vi "niRFSTS Digital Configure PPMU.vi"(0 "Semiconductor Module Context":T2, 3 "aperture time":dbl=4e-06 format="%#_6p", 4 "Level (V or A)":dbl, 5 "Pin Names":string[](array[string]), 9 "output function":T1=1300 items=["DC Voltage"=1300, "DC Current"=1301], 11 "error in (no error)":errorcluster, 12 "voltage limit high":dbl, 14 "voltage limit low":dbl) -> (15 "error out":errorcluster)   [LabVIEW 2014]
uses:
  <vilib>/NI_TestStand_SemiconductorModule/NI_TestStand_Semiconductor_Module.lvlibp/PinMap/General/SemiconductorModuleContext.ctl
  <instrlib>/niDigital/niDigital.llb/niDigital Output Function.ctl
  <instrlib>/niDigital/niDigital.llb/niDigital Selected Function.ctl
  <instrlib>/niDigital/niDigital.llb/niDigital PMU Aperture Time Units.ctl
  <vilib>/NI_TestStand_SemiconductorModule/NI_TestStand_Semiconductor_Module.lvlibp/PinMap/Digital Pattern/PinsToNIDigitalPatternSessions.vi
  <vilib>/NI_TestStand_SemiconductorModule/NI_TestStand_Semiconductor_Module.lvlibp
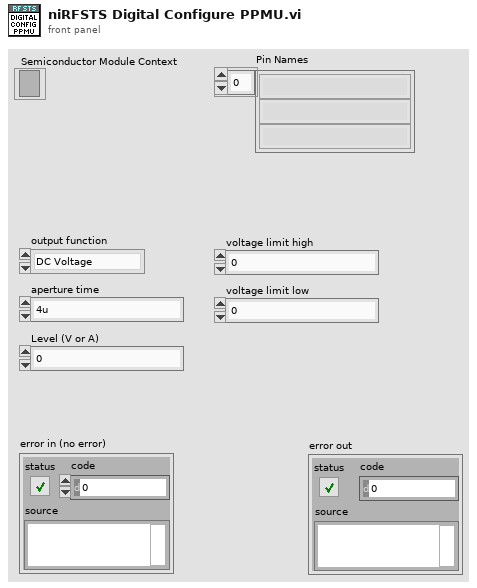
[diagram p1: front panel]
types:
  T1 = typedef "niDigital Output Function.ctl" = i32
  T2 = typedef "NI_TestStand_Semiconductor_Module.lvlibp/SemiconductorModuleContext.ctl" = refnum<k7>
  T3 = typedef "niDigital PMU Aperture Time Units.ctl" = i32
  T4 = typedef "niDigital Selected Function.ctl" = i32
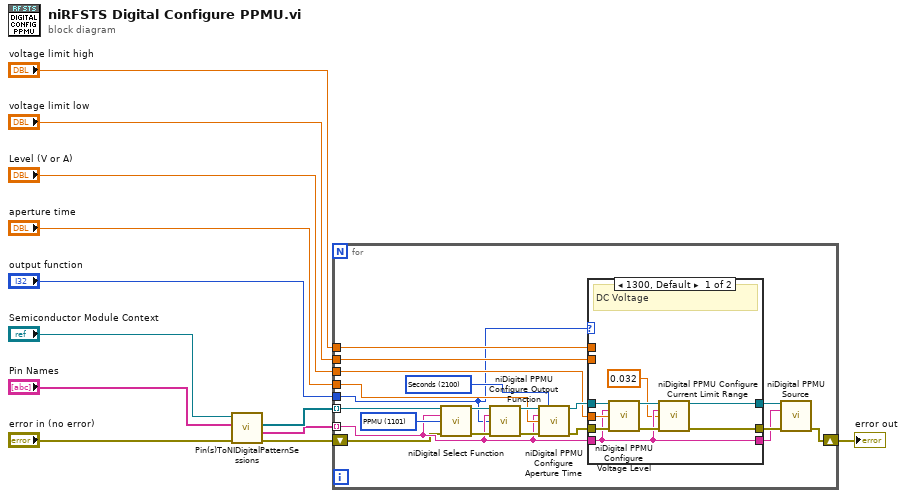
[diagram p0: block diagram]
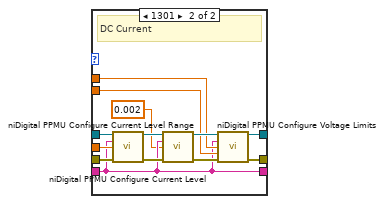
[diagram p2: hidden frame]
diagram:
  n1 = call-poly <vilib>:"Pin(s)ToNIDigitalPatternSessions.vi"("error in (no error)"="error in (no error)", "Pins"="Pin Names", "Semiconductor Module Context"="Semiconductor Module Context") -> ("error out"=w2:errorcluster, "Channel Lists"=w10:string[], "Instrument Sessions"=w11:refnum<k15>[])  [unwired: 3 in, 3 out]
  n2 = for {
    tunnel: w11 -> [w19] mode=indexing
    tunnel: w10 -> [w20] mode=indexing
    tunnel: "output function" -> [w13]
    tunnel: "Level (V or A)" -> [w25]
    tunnel: "voltage limit high" -> [w24]
    tunnel: "voltage limit low" -> [w23]
    tunnel: "aperture time" -> [w22]
    shift-right: [w16] -> w1
    shift-left: w2 -> [w18]
    w21 = T3 2100 items=["Seconds"=2100] ("aperture time units")
    w32 = T4 1101 items=["Digital"=1100, "PPMU"=1101, "Off"=1102, "Disconnect"=1103] ("function")
    n3 = call <instrlib>:"niDigital Select Function.vi"("instrument handle"=w19, "channel list"=w20, "function"=w32, "error in"=w18) -> ("instrument handle out"=w31:refnum<k15>, "error out"=w30:errorcluster)  [unwired: 10 in]
    n4 = call <instrlib>:"niDigital PPMU Configure Output Function.vi"("instrument handle"=w31, "channel list"=w20, "output function"=w13, "error in"=w30) -> ("instrument handle out"=w26:refnum<k15>, "error out"=w29:errorcluster)  [unwired: 10 in]
    n5 = call <instrlib>:"niDigital PPMU Configure Aperture Time.vi"("instrument handle"=w26, "aperture time units"=w21, "channel list"=w20, "aperture time"=w22, "error in"=w29) -> ("instrument handle out"=w27:refnum<k15>, "error out"=w28:errorcluster)  [unwired: 9 in]
    n6 = case shown="1300, Default" w13 {
      tunnel: w28 -> [w41 w54]
      tunnel: [w39 w51] -> w17
      tunnel: w27 -> [w38 w50]
      tunnel: w20 -> [w35 w44]
      tunnel: w25 -> [w36 w47]
      tunnel: w24 -> [_ w46]
      tunnel: w23 -> [_ w45]
      tunnel: [w35 w44] -> w14
      tunnel: [w34 w43] -> w15
      frame 1300, Default {
        # "DC Voltage"
        n7 = call <instrlib>:"niDigital PPMU Configure Voltage Level.vi"("instrument handle"=w38, "channel list"=w35, "voltage level (V)"=w36, "error in"=w41) -> ("instrument handle out"=w37:refnum<k15>, "error out"=w40:errorcluster)  [unwired: 10 in]
        n8 = call <instrlib>:"niDigital PPMU Configure Current Limit Range.vi"("instrument handle"=w37, "channel list"=w35, "current limit range (A)"=0.032 ("current level range (A)"), "error in"=w40) -> ("instrument handle out"=w34:refnum<k15>, "error out"=w39:errorcluster)  [unwired: 10 in]
      }
      frame 1301 {
        # "DC Current"
        n9 = call <instrlib>:"niDigital PPMU Configure Current Level.vi"("instrument handle"=w50, "channel list"=w44, "current level (A)"=w47, "error in"=w54) -> ("instrument handle out"=w49:refnum<k15>, "error out"=w53:errorcluster)  [unwired: 10 in]
        n10 = call <instrlib>:"niDigital PPMU Configure Current Level Range.vi"("instrument handle"=w49, "channel list"=w44, "current level range (A)"=0.002, "error in"=w53) -> ("instrument handle out"=w48:refnum<k15>, "error out"=w52:errorcluster)  [unwired: 10 in]
        n11 = call <instrlib>:"niDigital PPMU Configure Voltage Limits.vi"("instrument handle"=w48, "channel list"=w44, "voltage limit high (V)"=w46, "voltage limit low (V)"=w45, "error in"=w52) -> ("instrument handle out"=w43:refnum<k15>, "error out"=w51:errorcluster)  [unwired: 9 in]
      }
    }
    n12 = call <instrlib>:"niDigital PPMU Source.vi"("instrument handle"=w15, "channel list"=w14, "error in"=w17) -> ("error out"=w16:errorcluster)  [unwired: 11 in, 1 out]
  }
  "error out" <- w1
